vi "write camera settings.vi"(3 "Camera settings":T2={"Pixel format"=1, "exposure time [microsec]"=20.0, "Exposure time setting"=1, "gain [dB]"=0.0, "Auto Gain"=1, "Gamma enable"=FALSE, "gamma "=0.25, "ISP enable "=FALSE, "black level clamping enabled"=FALSE, "black level (%)"=0.0, "binning vertical"=1, "binning hor"=1, "vertical binning mode"=1, "horizontal  binning mode"=1, "width"=8.0, "height "=4.0} {"height" min=0.0 max=0.0 step=4.0; "width" min=0.0 max=0.0 step=4.0; "horizontal  binning mode" items=["Additive", "Average"]; "vertical binning mode" items=["Additive", "Average"]; "binning hor" items=["1", "2", "4"]; "binning vertical" items=["1", "2", "4"]; "black level (%)" min=-5.0 max=10.0; "gamma" min=0.25 max=4.0 step=0.1; "Auto Gain" items=["Continuous", "Once", "Off"]; "gain [dB]" min=0.0 max=47.0; "Exposure time setting" items=["Continuous", "Once", "Off"]; "exposure time [microsec]" min=20.0 max=30000000.0; "Pixel format" items=["Mono8", "Mono16", "Mono10Packed", "Mono12Packed", "Mono10p", "Mono12p"]}, 4 "error in":errorcluster, 5 "camera session  in":T1) -> (1 "error out":errorcluster, 2 "camera session out":T1)   [LabVIEW 2018]
uses:
  <vilib>/userdefined/High Color/IMAQdx.ctl
  <resource>/objmgr/imaqdx.rc
  <vilib>/vision/driver/NI_Vision_Acquisition_Software.lvlib
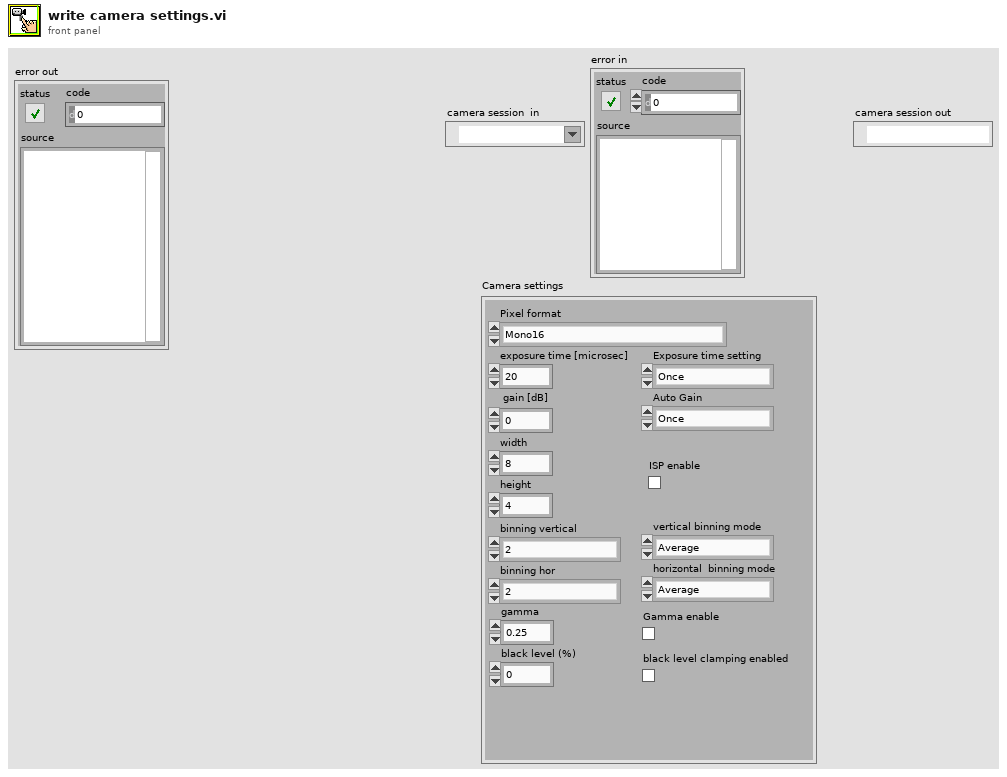
[diagram p1: front panel]
types:
  T1 = typedef "IMAQdx.ctl" = refnum<k21>
  T2 = cluster{"Pixel format":u16, "exposure time [microsec]":dbl, "Exposure time setting":u16, "gain [dB]":dbl, "Auto Gain":u16, "Gamma enable":bool, "gamma ":dbl, "ISP enable ":bool, "black level clamping enabled":bool, "black level (%)":dbl, "binning vertical":u16, "binning hor":u16, "vertical binning mode":u16, "horizontal  binning mode":u16, "width":dbl, "height ":dbl}
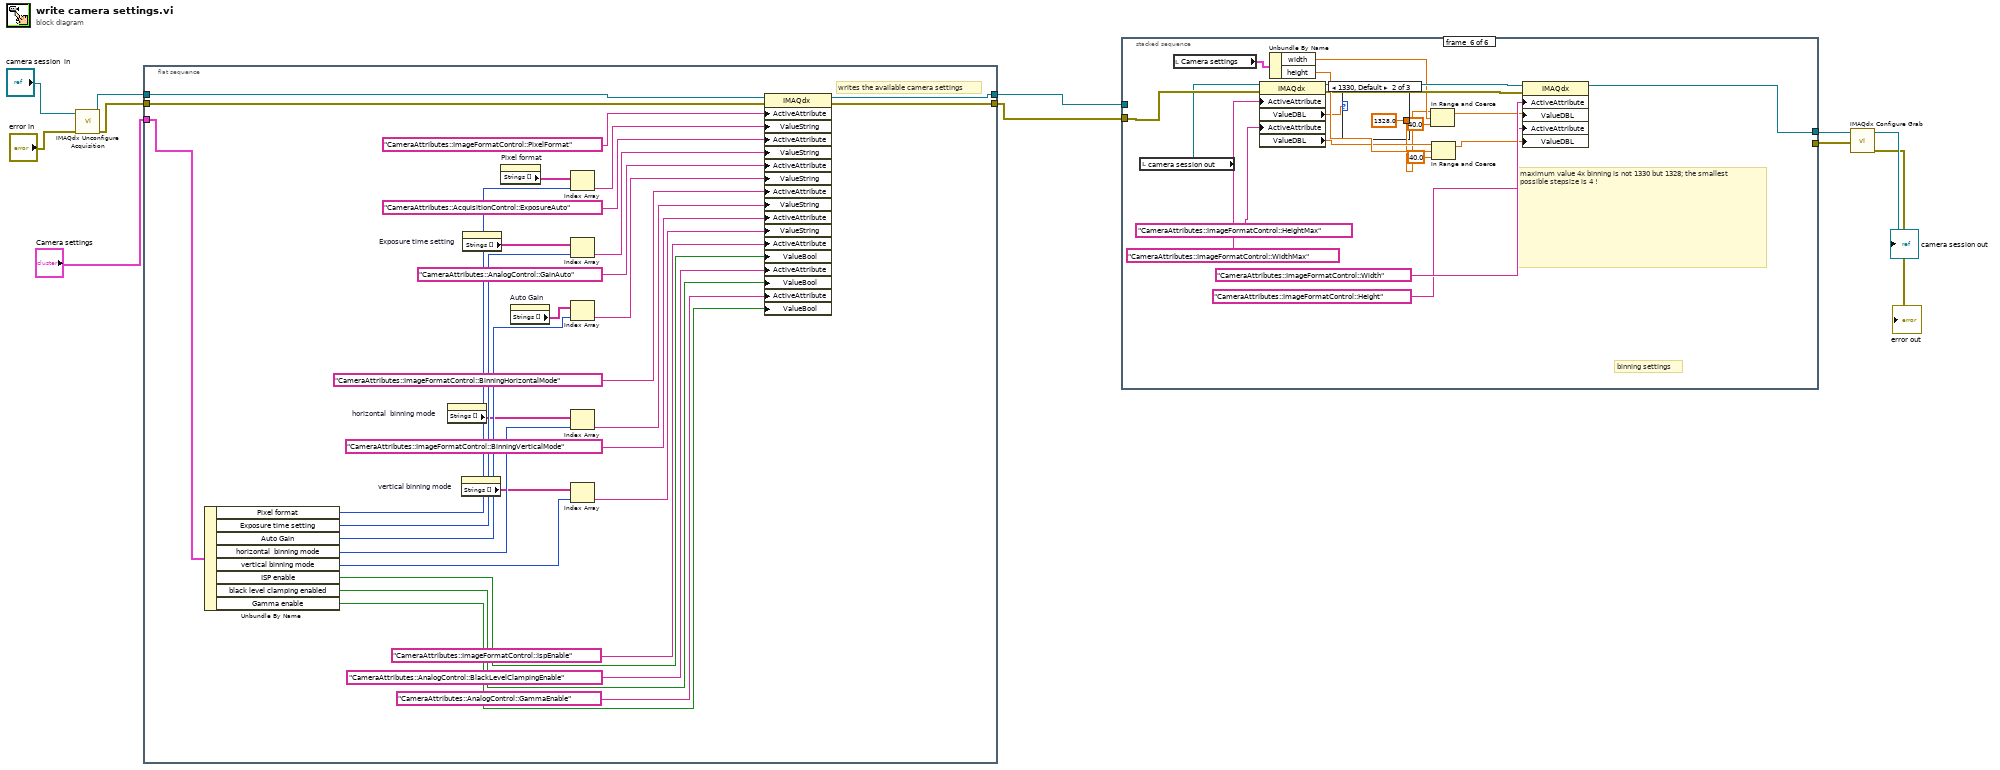
[diagram p0: block diagram]
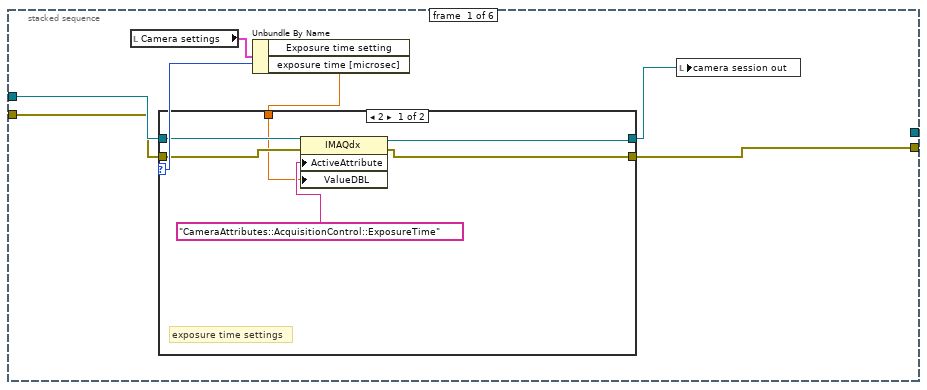
[diagram p2: hidden frame]
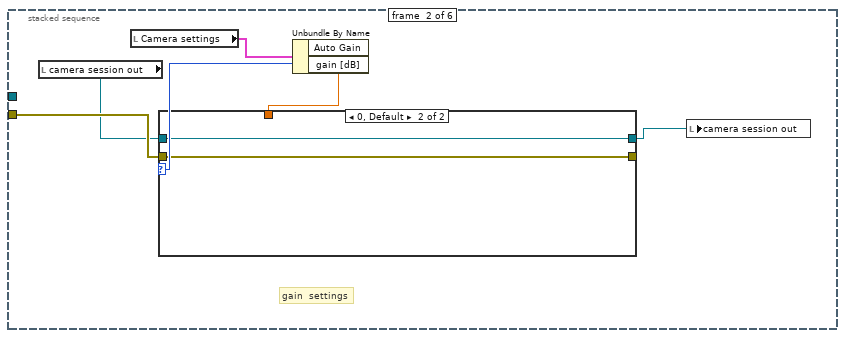
[diagram p4: hidden frame]
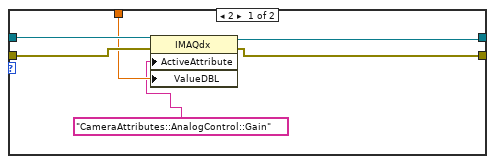
[diagram p5: hidden frame]
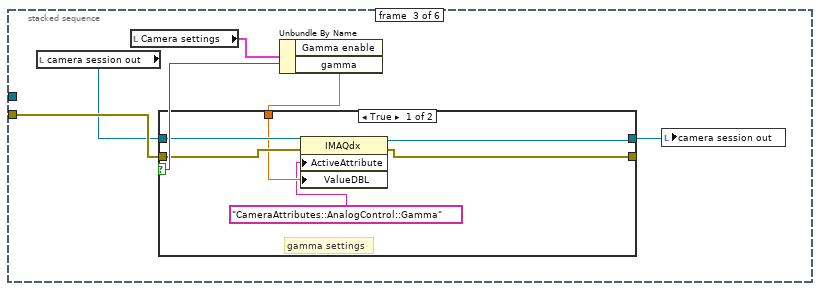
[diagram p6: hidden frame]
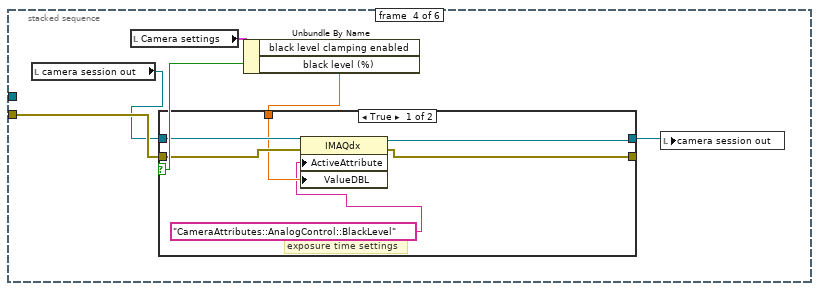
[diagram p8: hidden frame]
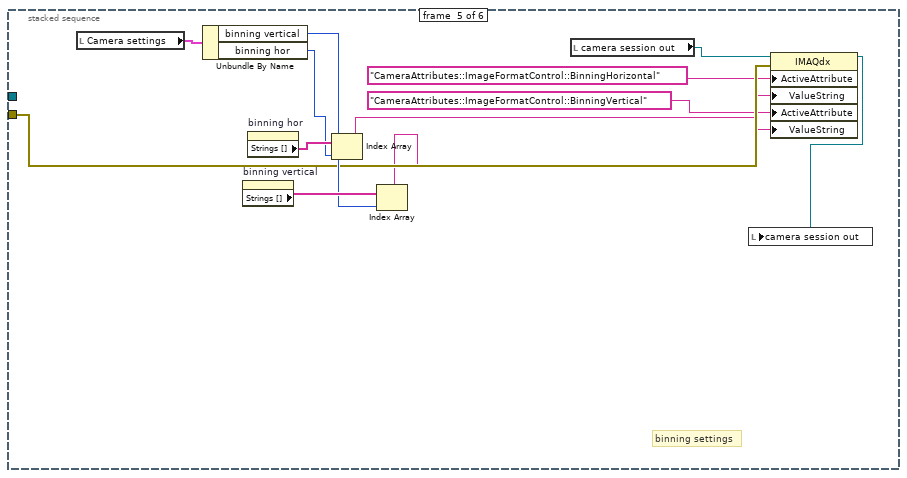
[diagram p10: hidden frame]
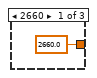
[diagram p11: hidden frame]
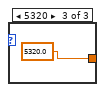
[diagram p12: hidden frame]
diagram:
  n1 = call <vilib>:"IMAQdx Unconfigure Acquisition.vi"("error in"="error in", "Session In"="camera session  in") -> ("error out"=w5:errorcluster, "Session Out"=w6:T1)  [unwired: 8 in]
  n2 = flat-sequence {
    tunnel: w6 -> [w42]
    tunnel: w5 -> [w41]
    tunnel: [w33] -> w11
    tunnel: [w32] -> w10
    tunnel: "Camera settings" -> [w13]
    frame #0 {
      # "writes the available camera settings"
      n3 = Unbundle By Name(w13) -> ("Pixel format"=w30:u16, "Exposure time setting"=w27:u16, "Auto Gain"=w24:u16, "horizontal  binning mode"=w19:u16, "vertical binning mode"=w16:u16, "ISP enable"=w14:bool, "black level clamping enabled"=w21:bool, "Gamma enable"=w22:bool)
      n4 = property on="horizontal  binning mode" class="Ring (strict)"() -> ("Strings []"=w20:string[])  [unwired: 2 in, 2 out]
      n5 = property on="vertical binning mode" class="Ring (strict)"() -> ("Strings []"=w17:string[])  [unwired: 2 in, 2 out]
      n6 = property on="Exposure time setting" class="Ring (strict)"() -> ("Strings []"=w28:string[])  [unwired: 2 in, 2 out]
      n7 = property on="Pixel format" class="Ring (strict)"() -> ("Strings []"=w31:string[])  [unwired: 2 in, 2 out]
      n8 = property on="Auto Gain" class="Ring (strict)"() -> ("Strings []"=w25:string[])  [unwired: 2 in, 2 out]
      n9 = Index Array(array=w31, index=w30) -> (element=w29:string)
      n10 = Index Array(array=w28, index=w27) -> (element=w26:string)
      n11 = Index Array(array=w25, index=w24) -> (element=w23:string)
      n12 = Index Array(array=w20, index=w19) -> (element=w18:string)
      n13 = Index Array(array=w17, index=w16) -> (element=w15:string)
      n14 = property class="IMAQdx"(reference=w42, error in=w41, "ActiveAttribute"="CameraAttributes::ImageFormatControl::PixelFormat", "ValueString"=w29, "ActiveAttribute"="CameraAttributes::AcquisitionControl::ExposureAuto", "ValueString"=w26, "ActiveAttribute"="CameraAttributes::AnalogControl::GainAuto", "ValueString"=w23, "ActiveAttribute"="CameraAttributes::ImageFormatControl::BinningHorizontalMode", "ValueString"=w18, "ActiveAttribute"="CameraAttributes::ImageFormatControl::BinningVerticalMode", "ValueString"=w15, "ActiveAttribute"="CameraAttributes::ImageFormatControl::IspEnable", "ValueBool"=w14, "ActiveAttribute"="CameraAttributes::AnalogControl::BlackLevelClampingEnable", "ValueBool"=w21, "ActiveAttribute"="CameraAttributes::AnalogControl::GammaEnable", "ValueBool"=w22) -> (reference out=w33:T1, error out=w32:errorcluster)
    }
  }
  n15 = stacked-sequence {
    tunnel: w11 -> [w48 _ _ _ _ _]
    tunnel: w10 -> [w47 w62 w76 w90 w106 w129]
    tunnel: [w46 _ _ _ _ _] -> w4
    tunnel: [_ _ _ _ _ w121] -> w1
    frame #0 {
      n16 = local read "Camera settings"() -> (w45:T2)
      n17 = Unbundle By Name(w45) -> ("Exposure time setting"=w49:u16, "exposure time [microsec]"=w44:dbl)
      n18 = case shown="2" w49 {
        tunnel: w48 -> [w55 w57]
        tunnel: w47 -> [w54 w56]
        tunnel: [w53 w57] -> w43
        tunnel: [w52 w56] -> w46
        tunnel: w44 -> [w50 _]
        frame 2 {
          # "exposure time settings"
          n19 = property class="IMAQdx"(reference=w55, error in=w54, "ActiveAttribute"="CameraAttributes::AcquisitionControl::ExposureTime", "ValueDBL"=w50) -> (reference out=w53:T1, error out=w52:errorcluster)
        }
        frame 0, Default {
        }
      }
      n20 = local write "camera session out"(w43) -> ()
    }
    frame #1 {
      # "gain  settings"
      n21 = local read "camera session out"() -> (w59:T1)
      n22 = local read "Camera settings"() -> (w61:T2)
      n23 = Unbundle By Name(w61) -> ("Auto Gain"=w63:u16, "gain [dB]"=w60:dbl)
      n24 = case shown="0, Default" w63 {
        tunnel: w59 -> [w69 w71]
        tunnel: w62 -> [w68 w70]
        tunnel: [w67 w71] -> w58
        tunnel: [w66 w70] -> _
        tunnel: w60 -> [w65 _]
        frame 2 {
          n25 = property class="IMAQdx"(reference=w69, error in=w68, "ActiveAttribute"="CameraAttributes::AnalogControl::Gain", "ValueDBL"=w65) -> (reference out=w67:T1, error out=w66:errorcluster)
        }
        frame 0, Default {
        }
      }
      n26 = local write "camera session out"(w58) -> ()
    }
    frame #2 {
      # "gamma settings"
      n27 = local read "camera session out"() -> (w73:T1)
      n28 = local read "Camera settings"() -> (w75:T2)
      n29 = Unbundle By Name(w75) -> ("Gamma enable"=w77:bool, "gamma"=w74:dbl)
      n30 = case shown="True" w77 {
        tunnel: w73 -> [w83 w85]
        tunnel: w76 -> [w82 w84]
        tunnel: [w81 w85] -> w72
        tunnel: [w80 w84] -> _
        tunnel: w74 -> [w79 _]
        frame True {
          n31 = property class="IMAQdx"(reference=w83, error in=w82, "ActiveAttribute"="CameraAttributes::AnalogControl::Gamma", "ValueDBL"=w79) -> (reference out=w81:T1, error out=w80:errorcluster)
        }
        frame False {
        }
      }
      n32 = local write "camera session out"(w72) -> ()
    }
    frame #3 {
      # "exposure time settings"
      n33 = local read "camera session out"() -> (w87:T1)
      n34 = local read "Camera settings"() -> (w89:T2)
      n35 = Unbundle By Name(w89) -> ("black level clamping enabled"=w91:bool, "black level (%)"=w88:dbl)
      n36 = case shown="True" w91 {
        tunnel: w87 -> [w97 w99]
        tunnel: w90 -> [w96 w98]
        tunnel: [w95 w99] -> w86
        tunnel: [w94 w98] -> _
        tunnel: w88 -> [w93 _]
        frame True {
          n37 = property class="IMAQdx"(reference=w97, error in=w96, "ActiveAttribute"="CameraAttributes::AnalogControl::BlackLevel", "ValueDBL"=w93) -> (reference out=w95:T1, error out=w94:errorcluster)
        }
        frame False {
        }
      }
      n38 = local write "camera session out"(w86) -> ()
    }
    frame #4 {
      # "binning settings"
      n39 = local read "Camera settings"() -> (w111:T2)
      n40 = Unbundle By Name(w111) -> ("binning vertical"=w107:u16, "binning hor"=w109:u16)
      n41 = property on="binning vertical" class="Ring (strict)"() -> ("Strings []"=w108:string[])  [unwired: 2 in, 2 out]
      n42 = property on="binning hor" class="Ring (strict)"() -> ("Strings []"=w110:string[])  [unwired: 2 in, 2 out]
      n43 = Index Array(array=w110, index=w109) -> (element=w105:string)
      n44 = Index Array(array=w108, index=w107) -> (element=w104:string)
      n45 = local read "camera session out"() -> (w101:T1)
      n46 = property class="IMAQdx"(reference=w101, error in=w106, "ActiveAttribute"="CameraAttributes::ImageFormatControl::BinningHorizontal", "ValueString"=w105, "ActiveAttribute"="CameraAttributes::ImageFormatControl::BinningVertical", "ValueString"=w104) -> (reference out=w100:T1)  [unwired: 1 out]
      n47 = local write "camera session out"(w100) -> ()
    }
    frame #5 {
      # "maximum value 4x binning is not 1330 but 1328; the smallest possible stepsize is 4 !"
      # "binning settings"
      n48 = local read "camera session out"() -> (w128:T1)
      n49 = local read "Camera settings"() -> (w130:T2)
      n50 = property class="IMAQdx"(reference=w128, error in=w129, "ActiveAttribute"="CameraAttributes::ImageFormatControl::WidthMax", "ActiveAttribute"="CameraAttributes::ImageFormatControl::HeightMax") -> (reference out=w123:T1, error out=w122:errorcluster, "ValueDBL"=w113:dbl, "ValueDBL"=w124:dbl)
      n51 = Unbundle By Name(w130) -> ("width"=w114:dbl, "height"=w125:dbl)
      n52 = case shown="1330, Default" w113 {
        tunnel: [2660.0 ("upper limit") 1328.0 ("upper limit") 5320.0 ("upper limit")] -> w112
        frame 2660 {
        }
        frame 1330, Default {
        }
        frame 5320 {
        }
      }
      n53 = In Range and Coerce(upper limit=w112, x=w114, lower limit=40.0) -> (coerced(x)=w118:dbl)  [unwired: 1 out]
      n54 = In Range and Coerce(upper limit=w124, x=w125, lower limit=40.0) -> (coerced(x)=w117:dbl)  [unwired: 1 out]
      n55 = property class="IMAQdx"(reference=w123, error in=w122, "ActiveAttribute"="CameraAttributes::ImageFormatControl::Width", "ValueDBL"=w118, "ActiveAttribute"="CameraAttributes::ImageFormatControl::Height", "ValueDBL"=w117) -> (reference out=w121:T1)  [unwired: 1 out]
    }
  }
  n56 = call <vilib>:"IMAQdx Configure Grab.vi"("error in"=w4, "Session In"=w1) -> ("error out"=→"error out":errorcluster, "Session Out"=→"camera session out":T1)  [unwired: 8 in]
